vi "Duplicate Folder with New Keyword.vi"() -> ()   [LabVIEW 2011]
doc: "This VI was provided by the Systems Engineering group at NI and signigicantly streamlines the process for creating a new set of VIs from a template. It serves as a classic example of a CASE tool that an archtiect would provide to a team of developers.\n\nAAL 9/09"
panel:
  out "error out":errorcluster
  in  "error in (no error)":errorcluster
  in  "New Keyword":string="Wind Turbine"
  in  "Destination Path":path=path "C:/Exercises/Advanced Architectures in LabVIEW/By Reference Objects/SEQ Wind Turbine Object"
  in  "Cancel":bool
  in  "ok":bool
  in  "Keyword to Replace":string="SEQ"
  in  "Root Path":path=path "C:/Exercises/Advanced Architectures in LabVIEW/By Reference Objects/SEQueue - Templates"
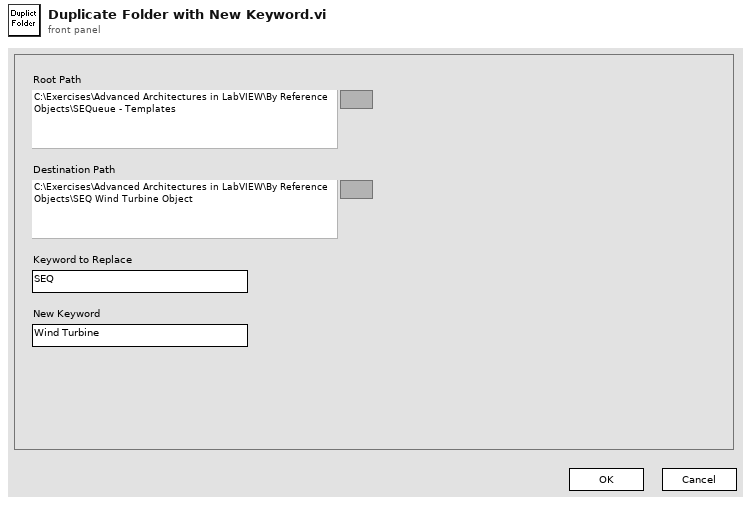
[diagram p1: front panel]
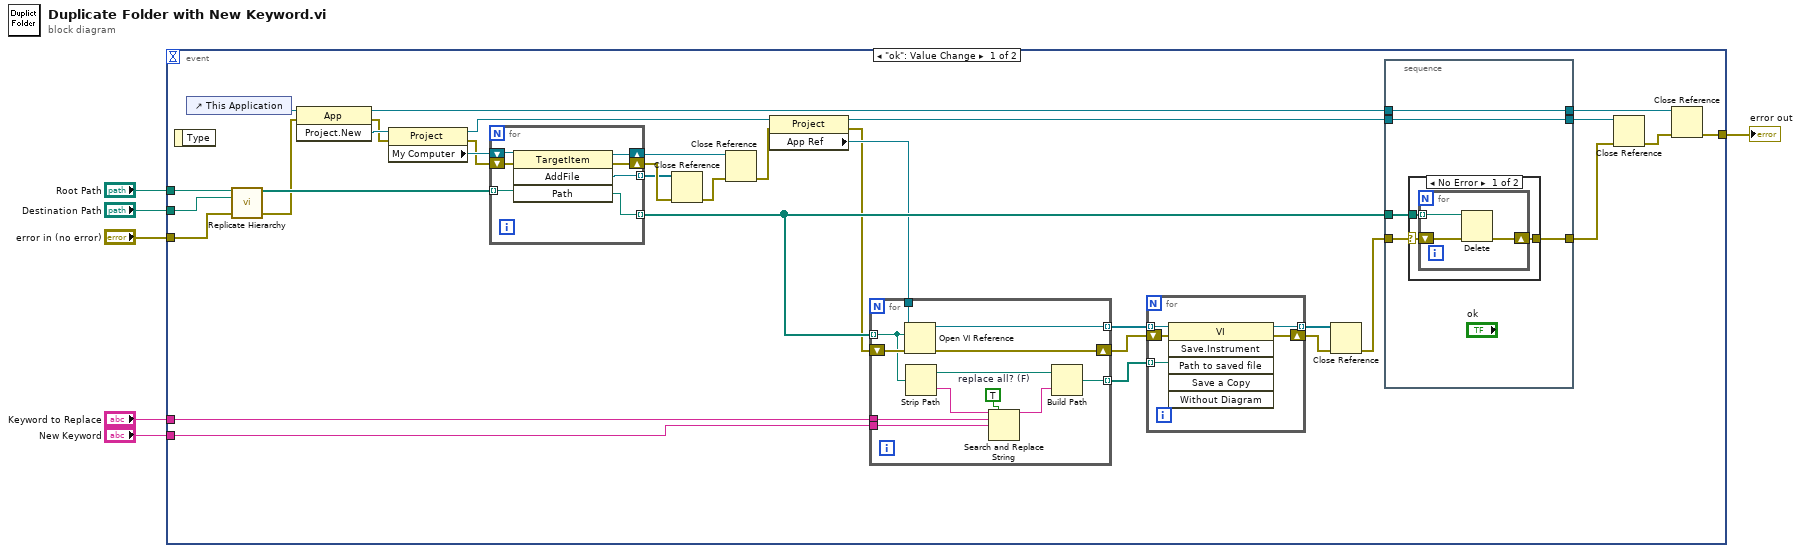
[diagram p0: block diagram]
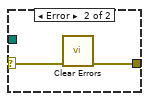
[diagram p2: hidden frame]
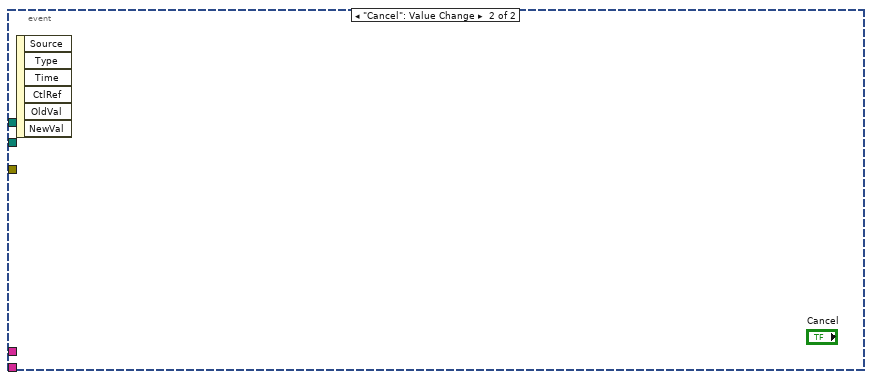
[diagram p3: hidden frame]
diagram:
  n1 = event shown="[0] \"ok\": Value Change" {
    selector: _ -> [_ _]
    dyn-events: _ -> [_ _]
    timeout: _ -> [_ _]
    tunnel: "Root Path" -> [w27 _]
    tunnel: "Destination Path" -> [w25 _]
    tunnel: "Keyword to Replace" -> [w33 _]
    tunnel: "New Keyword" -> [w32 _]
    tunnel: "error in (no error)" -> [w26 _]
    tunnel: [w15 _] -> w1
    event "ok": Value Change {
      n2 = event-data() -> ()  [unwired: 2 out]
      n3 = control-ref of="This Application"() -> (w39:refnum<vi>)
      n4 = call "Replicate Hierarchy.vi"("Root Path"=w27, "Destination Path"=w25, "error in (no error)"=w26) -> ("Replicated Hierarchy"=w28:path[], "error out"=w24:errorcluster)  [unwired: 5 in, 6 out]
      n5 = invoke class="App" method="Project.New"(reference=w39, error in=w24) -> (reference out=w36:refnum<vi>, error out=w23:errorcluster, "Project:New"=w37:refnum<vi>)  [unwired: 1 in]
      n6 = property class="Project"(reference=w37, error in=w23) -> (reference out=w10:refnum<vi>, error out=w22:errorcluster, "My Computer"=w38:refnum<vi>)
      n7 = for {
        tunnel: w28 -> [w74] mode=indexing
        tunnel: [w75] -> w35 mode=indexing
        tunnel: [w74] -> w29 mode=indexing
        shift-right: [w73] -> w30
        shift-left: w38 -> [w76]
        shift-right: [w71] -> w40
        shift-left: w22 -> [w72]
        n8 = invoke class="TargetItem" method="AddFile"(reference=w76, error in=w72, "Path"=w74) -> (reference out=w73:refnum<vi>, error out=w71:errorcluster, "AddFile"=w75:refnum<vi>)  [unwired: 1 in, 1 out]
      }
      n9 = Close Reference(reference=w35, error in (no error)=w40) -> (error out=w21:errorcluster)
      n10 = Close Reference(reference=w30, error in (no error)=w21) -> (error out=w9:errorcluster)
      n11 = property class="Project"(reference=w10, error in=w9) -> (reference out=w7:refnum<vi>, error out=w8:errorcluster, "App Ref"=w11:refnum<vi>)
      n12 = for {
        tunnel: w29 -> [w55] mode=indexing
        tunnel: [w56] -> w34 mode=indexing
        tunnel: w33 -> [w52]
        tunnel: w32 -> [w51]
        tunnel: [w48] -> w31 mode=indexing
        shift-right: [w47] -> w20
        shift-left: w8 -> [w57]
        tunnel: w11 -> [w46]
        w50 = TRUE  # replace all? (F)
        n13 = Open VI Reference(application reference (local)=w46, vi path=w55, error in (no error)=w57) -> (vi reference=w56:refnum<vi>, error out=w47:errorcluster)  [unwired: 3 out]
        n14 = Strip Path(path=w55) -> (stripped path=w54:path, name=w53:string)
        n15 = Search and Replace String(replace all?=w50, input string=w53, search string=w52, replace string=w51) -> (result string=w49:string)  [unwired: 1 in, 6 out]
        n16 = Build Path(base path=w54, name or relative path=w49) -> (appended path=w48:path)
      }
      n17 = for {
        tunnel: w34 -> [w45] mode=indexing
        tunnel: w31 -> [w44] mode=indexing
        shift-right: [w41] -> w13
        shift-left: w20 -> [w43]
        tunnel: [w42] -> w14 mode=indexing
        n18 = invoke class="VI" method="Save.Instrument"(reference=w45, error in=w43, "Path to saved file"=w44) -> (reference out=w42:refnum<vi>, error out=w41:errorcluster)  [unwired: 3 in, 4 out]
      }
      n19 = Close Reference(reference=w14, error in (no error)=w13) -> (error out=w12:errorcluster)
      n20 = stacked-sequence {
        tunnel: w36 -> [w59]
        tunnel: w7 -> [w58]
        tunnel: w29 -> [w62]
        tunnel: w12 -> [w61]
        tunnel: [w58] -> w19
        tunnel: [w59] -> w18
        tunnel: [w60] -> w16
        frame #0 {
          n21 = case shown="No Error" w61 {
            selector: w61 -> [w64 w70]
            tunnel: w62 -> [w65 _]
            tunnel: [w63 w69] -> w60
            frame No Error {
              n22 = for {
                tunnel: w65 -> [w68] mode=indexing
                shift-right: [w66] -> w63
                shift-left: w64 -> [w67]
                n23 = Delete(path (use dialog)=w68, error in=w67) -> (error out=w66:errorcluster)  [unwired: 5 out]
              }
            }
            frame Error {
              n24 = call <vilib>:"Clear Errors.vi"("error in (no error)"=w70) -> ("error out"=w69:errorcluster)  [unwired: 6 out]
            }
          }
        }
      }
      n25 = Close Reference(reference=w19, error in (no error)=w16) -> (error out=w17:errorcluster)
      n26 = Close Reference(reference=w18, error in (no error)=w17) -> (error out=w15:errorcluster)
    }
    event "Cancel": Value Change {
      n27 = event-data() -> ()  [unwired: 7 out]
    }
  }
  "error out" <- w1
